vi "tlc_Load.vi"(8 "error in (no error)":errorcluster, 10 "Path":path) -> (0 "error out":errorcluster)   [LabVIEW 2009]
doc: "[Covers: REQ_Load]\nImplements the Load functionality."
uses:
  Controls/tlc_User Interface Data Type.ctl
  Modules/Cue/tlc_Cue_Information Command.ctl
  Modules/File/tlc_File_Command Control.ctl
panel:
  # "Input"
  # "Output"
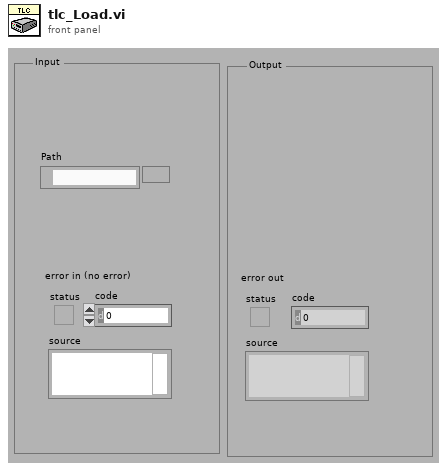
[diagram p1: front panel]
types:
  T1 = typedef "tlc_User Interface Data Type.ctl" = enum16{"Initialize", "Initialize Front Panel", "Update Front Panel Channels", "Select Cue in Cue List", "Enable/Disable Front Panel Controls", "Update Cue List", "Stop"}
  T2 = typedef "tlc_Cue_Information Command.ctl" = enum16{"Add Cue", "Get Cue Values", "Set Cue Values", "Get Number of Cues", "Initialize", "Get Empty Cue"}
  T3 = typedef "tlc_File_Command Control.ctl" = enum16{"Initialize", "Save Cues", "Load Cues", "Shutdown"}
  T4 = typedef "tlc_Cue_Information.ctl" = cluster{"Cue Name":string, "Wait Time (s)":u32, "Fade Time (s)":u32, "Follow Time (s)":u32, "Channels":T5[][]}
  T5 = typedef "channel.ctl" = cluster{"Intensity":dbl, " Color":u32, "Channel":i32}
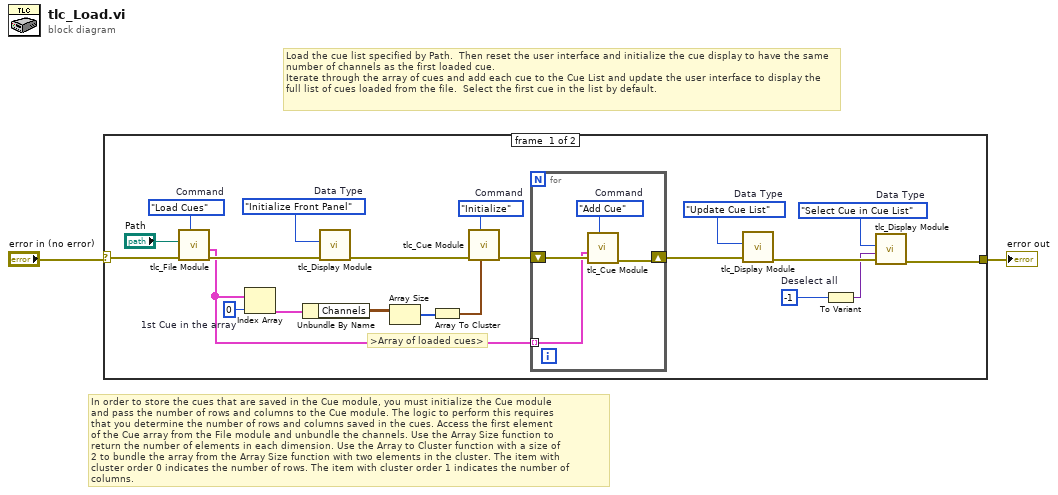
[diagram p0: block diagram]
diagram:
  # "In order to store the cues that are saved in the Cue module, you must initialize the Cue module \nand pass the number of rows and columns to the Cue module. The logic to perform this requires \nthat you determine the number of rows and columns saved in the cues. Access the first element \nof the Cue array from the File module and unbundle the channels. Use the Array Size function to \nreturn the number of elements in each dimension. Use the Array to Cluster function with a size of \n2 to bundle the array from the Array Size function with two elements in the cluster. The item with \ncluster order 0 indicates the number of rows. The item with cluster order 1 indicates the number of columns."
  # "Load the cue list specified by Path.  Then reset the user interface and initialize the cue display to have the same number of channels as the first loaded cue.\nIterate through the array of cues and add each cue to the Cue List and update the user interface to display the full list of cues loaded from the file.  Select the first cue in the list by default."
  n1 = case shown="No Error" "error in (no error)" {
    selector: "error in (no error)" -> [w23 w28]
    tunnel: [w6 w28] -> w1
    frame #0 {
      w5 = tlc_User_Interface_Data_Type."Select Cue in Cue List"  # Data Type
      w8 = tlc_User_Interface_Data_Type."Update Cue List"  # Data Type
      w17 = tlc_Cue_Information_Command."Initialize"  # Command
      w19 = tlc_User_Interface_Data_Type."Initialize Front Panel"  # Data Type
      w21 = tlc_File_Command_Control."Load Cues"  # Command
      w4 = -1  # Deselect all
      w16 = 0  # 1st Cue in the array
      # ">Array of loaded cues>"
      n2 = call "tlc_File Module.vi"("Command"=w21, "error in (no error)"=w23, "Path"="Path") -> ("error out"=w20:errorcluster, "Cue Array Output"=w10:T4[])  [unwired: 7 in]
      n3 = Index Array(array=w10, index=w16) -> (element=w15:T4)
      n4 = Unbundle By Name(w15) -> ("Channels"=w14:T5[][])
      n5 = call "tlc_Display Module.vi"("error in (no error)"=w20, "Data Type"=w19) -> ("error out"=w18:errorcluster)  [unwired: 9 in]
      n6 = Array Size(array=w14) -> (size(s)=w13:i32[])
      n7 = Array To Cluster(array=w13) -> (cluster=w12:cluster{"[0]":i32, "[1]":i32})
      n8 = call "tlc_Cue Module.vi"("Number of Channels"=w12, "Command"=w17, "error in (no error)"=w18) -> ("error out"=w11:errorcluster)  [unwired: 5 in, 2 out]
      n9 = for {
        shift-right: [w26] -> w9
        shift-left: w11 -> [w27]
        tunnel: w10 -> [w24] mode=indexing
        w25 = tlc_Cue_Information_Command."Add Cue"  # Command
        n10 = call "tlc_Cue Module.vi"("Command"=w25, "error in (no error)"=w27, "Cue Input"=w24) -> ("error out"=w26:errorcluster)  [unwired: 5 in, 2 out]
      }
      n11 = call "tlc_Display Module.vi"("error in (no error)"=w9, "Data Type"=w8) -> ("error out"=w7:errorcluster)  [unwired: 9 in]
      n12 = To Variant(anything=w4) -> (Variant=w3:variant)
      n13 = call "tlc_Display Module.vi"("error in (no error)"=w7, "Data"=w3, "Data Type"=w5) -> ("error out"=w6:errorcluster)  [unwired: 8 in]
    }
    frame #1 {
    }
  }
  "error out" <- w1
